vi "replaceConditionToken.vi"(8 "error in (no error)":errorcluster, 10 "Query In":string, 11 "Banking Transactions in":refnum<class "BankingTransactionList.lvclass">) -> (0 "error out":errorcluster, 2 "Query Out":string, 3 "Banking Transactions out":refnum<class "BankingTransactionList.lvclass">)   [LabVIEW 2018, in "BankingTransactionList.lvclass"]
uses:
  BankingTransactionList.lvclass
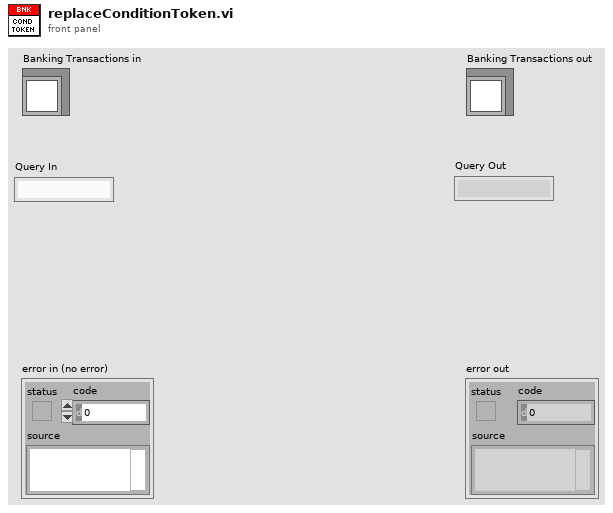
[diagram p1: front panel]
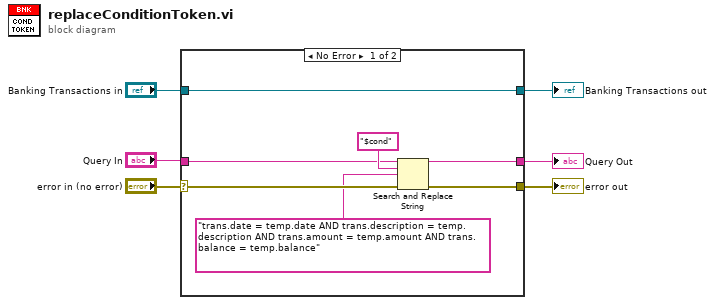
[diagram p0: block diagram]
diagram:
  n1 = case shown="No Error" "error in (no error)" {
    selector: "error in (no error)" -> [w8 w14]
    tunnel: [w10 w15] -> w5
    tunnel: "Query In" -> [w9 _]
    tunnel: "Banking Transactions in" -> [w10 w15]
    tunnel: [w13 w14] -> w4
    tunnel: [w12 _] -> w3
    frame No Error {
      n2 = Search and Replace String(input string=w9, search string="$cond", replace string="trans.date = temp.date AND trans.description = temp.description AND trans.amount = temp.amount AND trans.balance = temp.balance", error in=w8) -> (result string=w12:string, error out=w13:errorcluster)  [unwired: 4 in, 2 out]
    }
    frame Error {
    }
  }
  "error out" <- w4
  "Banking Transactions out" <- w5
  "Query Out" <- w3
